vi "Parse Builds.vi"(10 "Project Path":path=path "C:/dev/Vireo/PicoG/PicoG-Lib.lvproject") -> (2 "Builds":T1[](array[typedef]))   [LabVIEW 2020, in "PicoG-Processor.lvlib" / "WebProjectWatcher.lvclass"]
uses:
  WebProjectWatcher.lvclass
  Web Build.ctl
  <vilib>/xml/Load XML File.vi
  <vilib>/xml/Close Reference(Node).vi
  <vilib>/xml/NI_XML.lvlib
panel:
  out "Vireo Component Ids":string[](array[string])
  out "error out":errorcluster
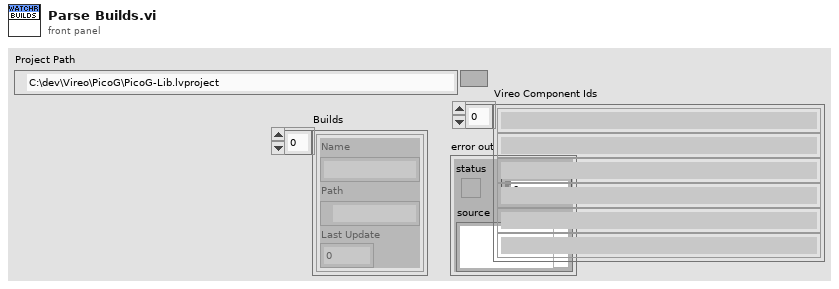
[diagram p1: front panel]
types:
  T1 = typedef "PicoG-Processor.lvlib/WebProjectWatcher.lvclass/Web Build.ctl" = cluster{"Name":string, "Path":path, "Last Update":dbl}
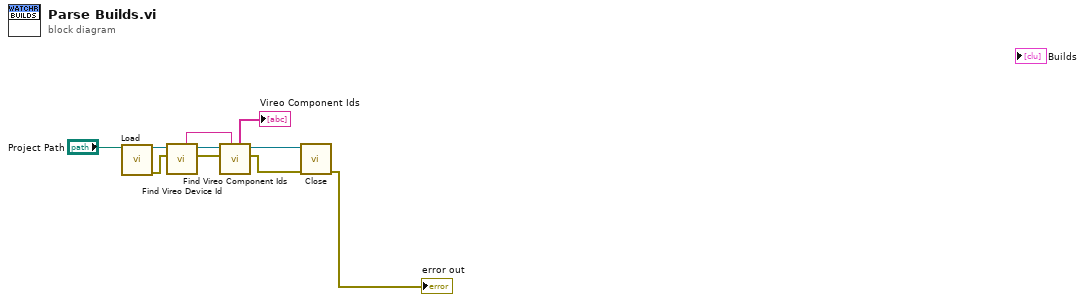
[diagram p0: block diagram]
diagram:
  n1 = call-poly <vilib>:"Load.vi"("path to XML document"="Project Path") -> ("DOM document out"=w8:refnum<k20>, "error out"=w9:errorcluster)  [unwired: 12 in, 1 out]
  n2 = call "Find Vireo Device Id.vi"("error in (no error)"=w9, "XML in"=w8) -> ("error out"=w5:errorcluster, "XML"=w6:refnum<k20>, "Vireo Target ID"=w4:string)  [unwired: 7 in]
  n3 = call "Find Vireo Component Ids.vi"("Vireo Target ID"=w4, "error in (no error)"=w5, "XML in"=w6) -> ("error out"=w1:errorcluster, "XML"=w2:refnum<k20>, "Vireo Component Ids"=→"Vireo Component Ids":string[])  [unwired: 6 in]
  n4 = call-poly <vilib>:"Close.vi"("error in (no error)"=w1, "node"=w2) -> ("error out"=→"error out":errorcluster)  [unwired: 7 in]
